vi "Remove System.vi"(8 "error in (no error)":errorcluster, 11 "Manager in":refnum<class "Manager.lvclass">) -> (0 "error out":errorcluster, 3 "Manager out":refnum<class "Manager.lvclass">)   [LabVIEW 2013, in "Manager.lvlib" / "Manager.lvclass"]
uses:
  Manager.lvclass
  Manager.lvclass/Manager.ctl
  Write Control Systems.vi
  Read System Ring Refnum.vi
  Read Control Systems.vi
  Read Remove Button Refnum.vi
  PluginInterface/Actor Framework.lvlibp/Message Enqueuer/Enqueue.vi
  PluginInterface/Actor Framework.lvlibp/Message Enqueuer/Message Enqueuer.lvclass
  Manager Messages/Update SubPanel Msg/Update SubPanel Msg.lvclass
  PluginInterface/Actor Framework.lvlibp/Stop Msg/Stop Msg.lvclass
  PluginInterface/Actor Framework.lvlibp/Actor/Actor.lvclass
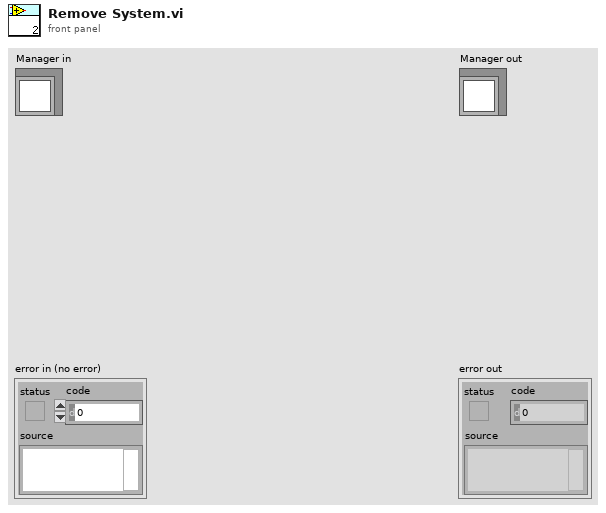
[diagram p1: front panel]
types:
  T1 = cluster{"Name":string, "Plugins":refnum<class "Message Enqueuer.lvclass">[]}[]
  T2 = cluster{"Name":string, "Plugins":refnum<class "Message Enqueuer.lvclass">[]}
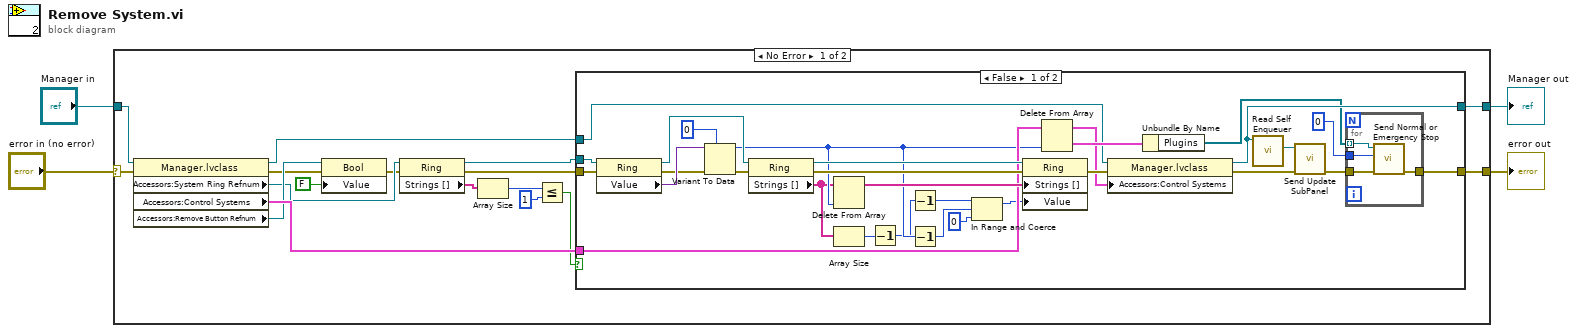
[diagram p0: block diagram]
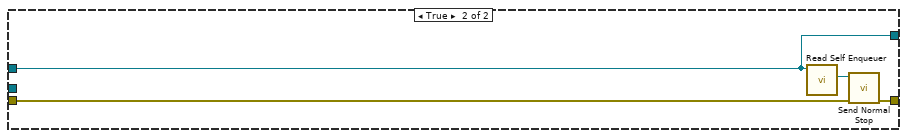
[diagram p2: hidden frame]
diagram:
  n1 = case shown="No Error" "error in (no error)" {
    selector: "error in (no error)" -> [w21 w61]
    tunnel: [w19 w61] -> w3
    tunnel: [w16 w60] -> w1
    tunnel: "Manager in" -> [w20 w60]
    frame No Error {
      n2 = property class="Manager.lvclass"(reference=w20, error in=w21) -> (reference out=w17:refnum<class "Manager.lvclass">, error out=w13:errorcluster, "Accessors:System Ring Refnum"=w12:refnum<vi>, "Accessors:Control Systems"=w18:T1, "Accessors:Remove Button Refnum"=w15:refnum<vi>)
      n3 = property class="Bool"(reference=w15, error in=w13, "Value"=FALSE) -> (error out=w10:errorcluster)  [unwired: 1 out]
      n4 = property class="Ring"(reference=w12, error in=w10) -> (reference out=w11:refnum<vi>, error out=w9:errorcluster, "Strings []"=w8:string[])
      n5 = Array Size(array=w8) -> (size(s)=w5:i32)
      n6 = Less Or Equal?(x=w5, y=1) -> (x <= y?=w6:bool)
      n7 = case shown="False" w6 {
        tunnel: [w40 w57] -> w19
        tunnel: w18 -> [w39 _]
        tunnel: w17 -> [w37 w56]
        tunnel: [w36 w56] -> w16
        tunnel: w11 -> [w32 _]
        tunnel: w9 -> [w31 w58]
        frame False {
          n8 = property class="Ring"(reference=w32, error in=w31) -> (reference out=w47:refnum<vi>, error out=w49:errorcluster, "Value"=w51:variant)
          n9 = Variant To Data(error in=w49, type=0, Variant=w51) -> (data=w30:i32, error out=w48:errorcluster)
          n10 = property class="Ring"(reference=w47, error in=w48) -> (reference out=w45:refnum<vi>, error out=w44:errorcluster, "Strings []"=w25:string[])
          n11 = Delete From Array(array=w25, index=w30) -> (array with subset deleted=w46:string[])  [unwired: 1 in, 1 out]
          n12 = Array Size(array=w25) -> (size(s)=w24:i32)
          n13 = Decrement(x=w24) -> (x-1=w29:i32)
          n14 = Decrement(x=w29) -> (x-1=w23:i32)
          n15 = Decrement(x=w30) -> (x-1=w27:i32)
          n16 = In Range and Coerce(upper limit=w23, x=w27, lower limit=0) -> (coerced(x)=w26:i32)  [unwired: 1 out]
          n17 = property class="Ring"(reference=w45, error in=w44, "Strings []"=w46, "Value"=w26) -> (error out=w35:errorcluster)  [unwired: 1 out]
          n18 = Delete From Array(array=w39, index=w30) -> (deleted portion=w38:T2, array with subset deleted=w33:T1)  [unwired: 1 in]
          n19 = property class="Manager.lvclass"(reference=w37, error in=w35, "Accessors:Control Systems"=w33) -> (reference out=w36:refnum<class "Manager.lvclass">, error out=w34:errorcluster)
          n20 = Unbundle By Name(w38) -> ("Plugins"=w22:refnum<class "Message Enqueuer.lvclass">[])
          n21 = call "Read Self Enqueuer.vi"("Actor"=w36) -> ("Self Enqueuer"=w42:refnum<class "Message Enqueuer.lvclass">)  [unwired: 10 in]
          n22 = call "Send Update SubPanel.vi"("error in (no error)"=w34, "Message Enqueuer"=w42) -> ("error out"=w41:errorcluster)  [unwired: 8 in, 1 out]
          n23 = for {
            tunnel: w22 -> [w55] mode=indexing
            tunnel: 0 ("final error code") -> [w54]
            tunnel: [w53] -> w40
            tunnel: w41 -> [w52]
            n24 = call "Send Normal or Emergency Stop.vi"("error in (no error)"=w52, "final error code"=w54, "Message Enqueuer"=w55) -> ("error out"=w53:errorcluster)  [unwired: 8 in]
          }
        }
        frame True {
          n25 = call "Read Self Enqueuer.vi"("Actor"=w56) -> ("Self Enqueuer"=w59:refnum<class "Message Enqueuer.lvclass">)  [unwired: 10 in]
          n26 = call "Send Normal Stop.vi"("error in (no error)"=w58, "Message Enqueuer"=w59) -> ("error out"=w57:errorcluster)  [unwired: 9 in]
        }
      }
    }
    frame Error {
    }
  }
  "error out" <- w3
  "Manager out" <- w1
